vi "Get End GPS Coordinate.vi"(1 "Bearing(Theta)":dbl, 2 "Distance":dbl, 3 "Start GPS coordinate":T1={"Latitude"=2504.69148, "Longitude"=4361.44351} {"Longitude" format="%#_14g"; "Latitude" format="%#_14g"}) -> (0 "End GPS coordinate":T1 {"Longitude" format="%#_14g"; "Latitude" format="%#_14g"})   [LabVIEW 2009]
uses:
  TypeDefs/Sensor TypeDefs/GPS Data.ctl
panel:
  out "Degrees":dbl
  # "In Radians"
  # "http://www.movable-type.co.uk/scripts/latlong.html"
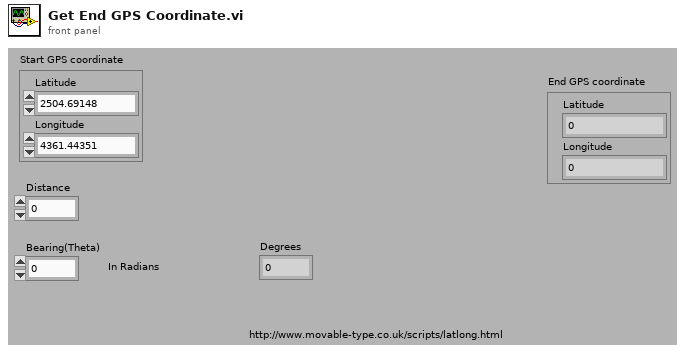
[diagram p1: front panel]
types:
  T1 = typedef "GPS Data.ctl" = cluster{"Latitude":dbl, "Longitude":dbl}
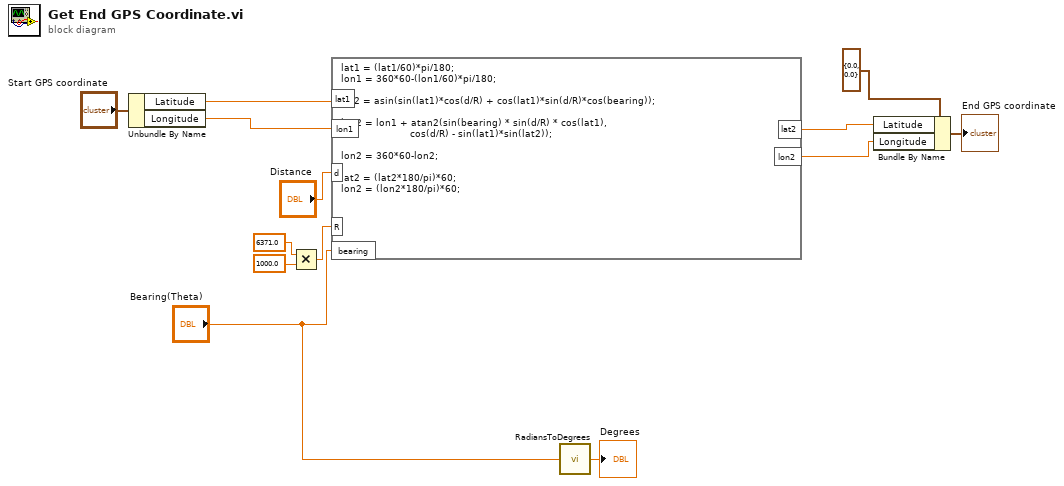
[diagram p0: block diagram]
diagram:
  n1 = Unbundle By Name("Start GPS coordinate") -> ("Latitude"=w6:dbl, "Longitude"=w5:dbl)
  n2 = Multiply(x=6371.0 ("Distance"), y=1000.0) -> (x*y=w7:dbl)
  n3 = formula code="lat1 = (lat1/60)*pi/180;\nlon1 = 360*60-(lon1/60)*pi/180;\n\nlat2 = asin(sin(lat1)*cos(d/R) + cos(lat1)*sin(d/R)*cos(bearing));\n\nlon2 = lon1 + atan2(sin(bearing) * sin(d/R) * cos(lat1), \n                       cos(d/R) - sin(lat1)*sin(lat2));\n\nlon2 = 360*60-lon2;\n\nlat2 = (lat2*180/pi)*60;\nlon2 = (lon2*180/pi)*60;"("lat1"=w6, "d"="Distance", "R"=w7, "bearing"="Bearing(Theta)", "lon1"=w5) -> ("lat2"=w4:dbl, "lon2"=w3:dbl)
  n4 = call "RadiansToDegrees.vi"("Radians"="Bearing(Theta)") -> ("Degrees"=→"Degrees":dbl)
  n5 = Bundle By Name(cluster=T1 {"Latitude"=0.0, "Longitude"=0.0} ("GPS Co-ordinates"), "Latitude"=w4, "Longitude"=w3) -> (→"End GPS coordinate":T1)
